vi "Check Status.vi"(8 "error in (no error)":errorcluster, 11 "Power Meter in":refnum<class "Power Meter.lvclass">) -> (0 "error out":errorcluster, 1 "Status":string, 2 "Ready?":bool, 3 "Power Meter out":refnum<class "Power Meter.lvclass">)   [LabVIEW 2017, in "Power Meter.lvclass"]
doc: "(Dynamic) Check if the instrument is powered on and update its member fields with the instrument's current status. Optionally return a text status message."
uses:
  Power Meter.lvclass
  Power Meter.lvclass/Power Meter.ctl
  Utility Classes/Readable/Readable.lvclass
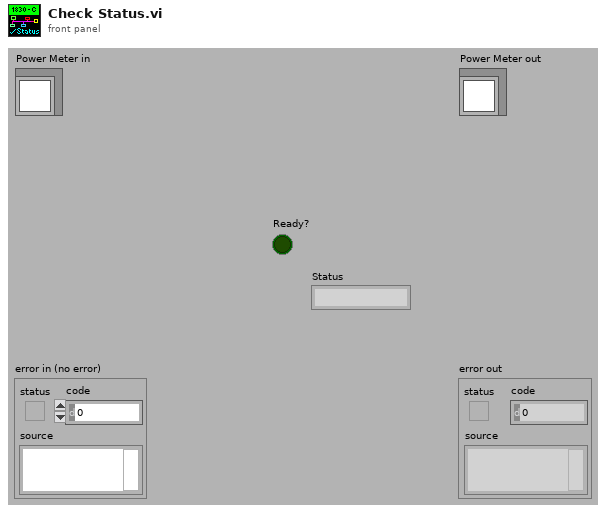
[diagram p1: front panel]
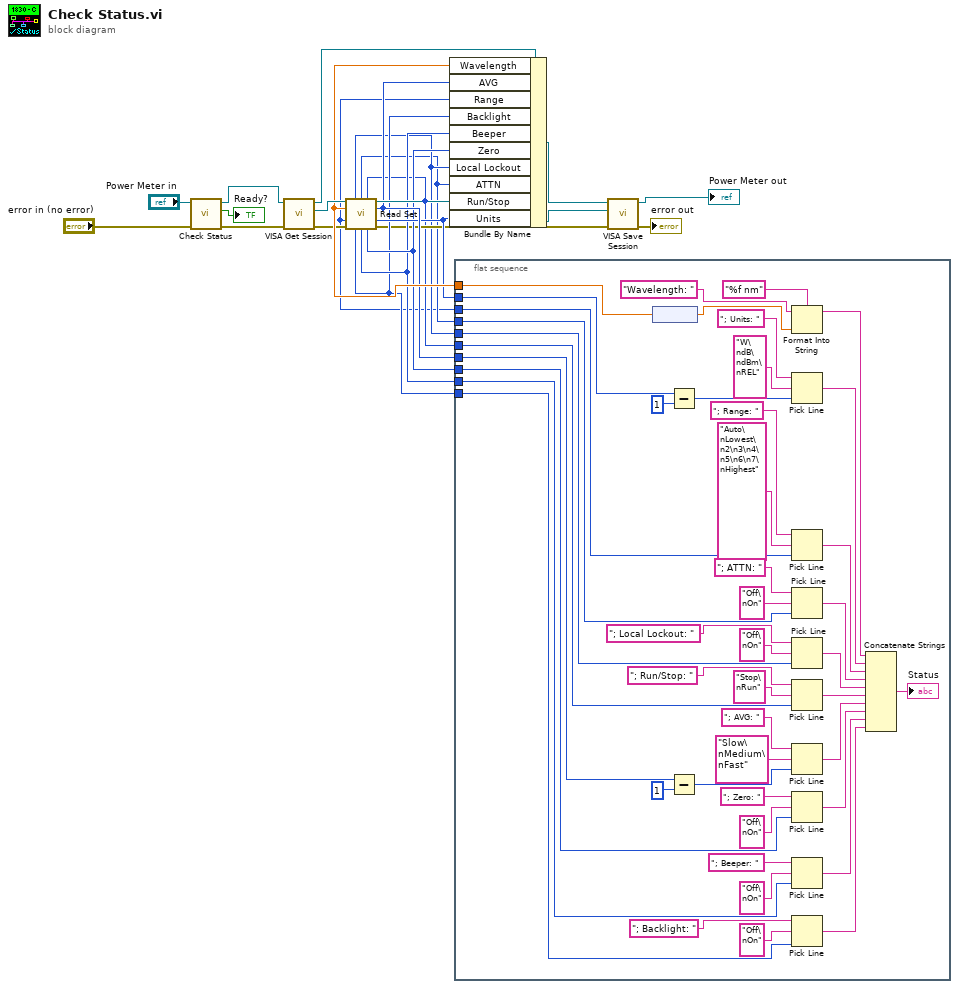
[diagram p0: block diagram]
diagram:
  n1 = call-parent "Check Status.vi"("error in (no error)"="error in (no error)", "Instrument in"="Power Meter in") -> ("error out"=w18:errorcluster, "Ready?"=→"Ready?":bool, "Instrument out"=w20:refnum<class "Power Meter.lvclass">)  [unwired: 6 in, 1 out]
  n2 = call-dynamic "VISA Get Session.vi"("error in (no error)"=w18, "Instrument.lvclass in"=w20) -> ("error out"=w6:errorcluster, "VISA Resource Name"=w14:refnum<visa-resource-name>, "Instrument.lvclass out"=w16:refnum<class "Power Meter.lvclass">)  [unwired: 7 out]
  n3 = call "Read Set.vi"("VISA resource name"=w14, "error in (no error)"=w6) -> ("Local Lockout"=w4:u32, "ATTN"=w3:u32, "Run/Stop"=w2:u32, "VISA resource name out"=w13:refnum<visa-resource-name>, "Wavelength (nnnn)"=w12:dbl[unit], "AVG"=w11:u32, "Range (1:8)"=w1:u32, "Units"=w10:u32, "Backlight"=w7:u32, "Beeper"=w8:u32, "Zero"=w9:u32, "error out"=w5:errorcluster)  [unwired: 2 in]
  n4 = Bundle By Name(cluster=w16, "Wavelength"=w12, "AVG"=w11, "Range"=w1, "Backlight"=w7, "Beeper"=w8, "Zero"=w9, "Local Lockout"=w4, "ATTN"=w3, "Run/Stop"=w2, "Units"=w10) -> (w15:refnum<class "Power Meter.lvclass">)
  n5 = flat-sequence {
    tunnel: w10 -> [w61]
    tunnel: w12 -> [w57]
    tunnel: w3 -> [w55]
    tunnel: w1 -> [w51]
    tunnel: w4 -> [w47]
    tunnel: w2 -> [w43]
    tunnel: w11 -> [w39]
    tunnel: w9 -> [w33]
    tunnel: w8 -> [w29]
    tunnel: w7 -> [w25]
    frame #0 {
      n6 = node(w57) -> (w69:dbl)
      n7 = Subtract(x=w61, y=u32 1) -> (x-y=w59:u32)
      n8 = Subtract(x=w39, y=u32 1) -> (x-y=w37:u32)
      n9 = Format Into String(format string="%f nm", initial string="Wavelength: ", w69) -> (resulting string=w64:string)  [unwired: 1 in, 1 out]
      n10 = Pick Line(string ("")="; Units: ", multi-line string="W\ndB\ndBm\nREL", line index=w59) -> (output string=w63:string)
      n11 = Pick Line(string ("")="; Range: ", multi-line string="Auto\nLowest\n2\n3\n4\n5\n6\n7\nHighest", line index=w51) -> (output string=w50:string)
      n12 = Pick Line(string ("")="; ATTN: ", multi-line string="Off\nOn", line index=w55) -> (output string=w54:string)
      n13 = Pick Line(string ("")="; Local Lockout: ", multi-line string="Off\nOn", line index=w47) -> (output string=w46:string)
      n14 = Pick Line(string ("")="; Run/Stop: ", multi-line string="Stop\nRun", line index=w43) -> (output string=w42:string)
      n15 = Pick Line(string ("")="; AVG: ", multi-line string="Slow\nMedium\nFast", line index=w37) -> (output string=w36:string)
      n16 = Pick Line(string ("")="; Zero: ", multi-line string="Off\nOn", line index=w33) -> (output string=w32:string)
      n17 = Pick Line(string ("")="; Beeper: ", multi-line string="Off\nOn", line index=w29) -> (output string=w28:string)
      n18 = Pick Line(string ("")="; Backlight: ", multi-line string="Off\nOn", line index=w25) -> (output string=w24:string)
      n19 = Concatenate Strings(w64, w63, w50, w54, w46, w42, w36, w32, w28, w24) -> (→"Status":string)
    }
  }
  n20 = call-dynamic "VISA Save Session.vi"("error in (no error)"=w5, "VISA Resource Name"=w13, "Instrument.lvclass in"=w15) -> ("error out"=→"error out":errorcluster, "Instrument.lvclass out"=→"Power Meter out":refnum<class "Power Meter.lvclass">)  [unwired: 7 out]
